vi "Write shared registers.vi"(10 "niInstr Instruction Framework Interfaces v1 FPGA.lvlib:Address Space Collection.lvclass":refnum<class "Address Space Collection.lvclass">, 11 "niUSRP Stream Control v1 FPGA.lvclass":refnum<class "niUSRP Sync v1 FPGA.lvclass">) -> (3 "niUSRP Stream Control v1 FPGA.lvclass 2":refnum<class "niUSRP Sync v1 FPGA.lvclass">)   [LabVIEW 2025, in "niUSRP Sync v1 FPGA.lvclass"]
uses:
  niUSRP Sync v1 FPGA.lvclass
  <instrlib>/_niInstr/Instruction Framework/v1/FPGA/Interfaces/Address Space Collection/Address Space Collection.lvclass
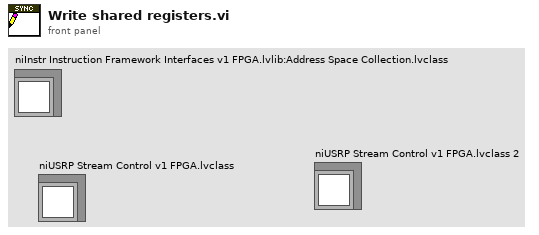
[diagram p1: front panel]
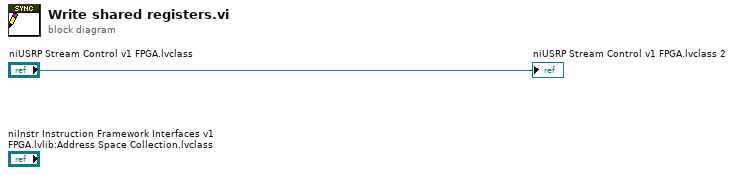
[diagram p0: block diagram]
diagram:
  "niUSRP Stream Control v1 FPGA.lvclass 2" <- "niUSRP Stream Control v1 FPGA.lvclass"
